vi "demo - first for loop.vi"() -> ()   [LabVIEW 2024]
doc: "#vi_description \nPlot a finite sine wave onto a waveform chart\nThetic Engineering Ltd."
panel:
  out "current iteration":i32
  out "Waveform Chart":dbl(graph)
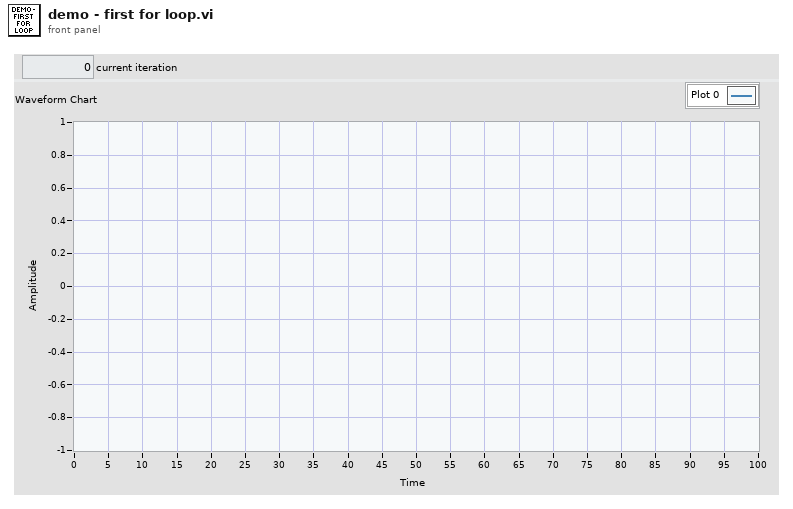
[diagram p1: front panel]
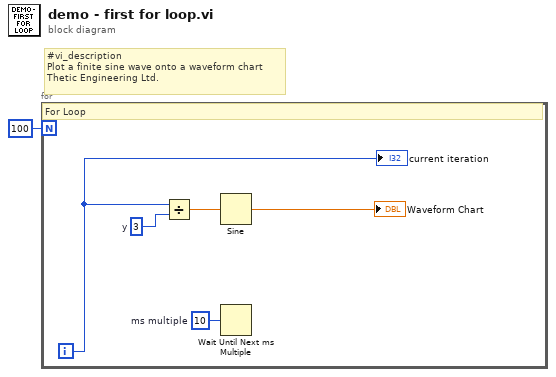
[diagram p0: block diagram]
diagram:
  # "#vi_description \nPlot a finite sine wave onto a waveform chart\nThetic Engineering Ltd."
  n1 = for {
    N: 100 -> [_]
    i -> [w2]
    w3 = u32 10  # ms multiple
    w4 = 3  # y
    # "For Loop"
    n2 = Divide(x=w2, y=w4) -> (x/y=w5:dbl)
    n3 = Sine(x=w5) -> (sin(x)=→"Waveform Chart":dbl)
    n4 = Wait Until Next ms Multiple(millisecond multiple=w3) -> ()  [unwired: 1 out]
    "current iteration" <- w2
  }
